vi "Initialise Front Panel.vi"(8 "error in (no error)":errorcluster, 11 "Actor in":refnum<class "Actor.lvclass">) -> (0 "error out":errorcluster, 3 "Actor out":refnum<class "Actor.lvclass">)   [LabVIEW 2015, in "Actor.lvclass"]
uses:
  Actor.lvclass
  Actor.lvclass/Actor.ctl
  Utility/Utility.lvlib
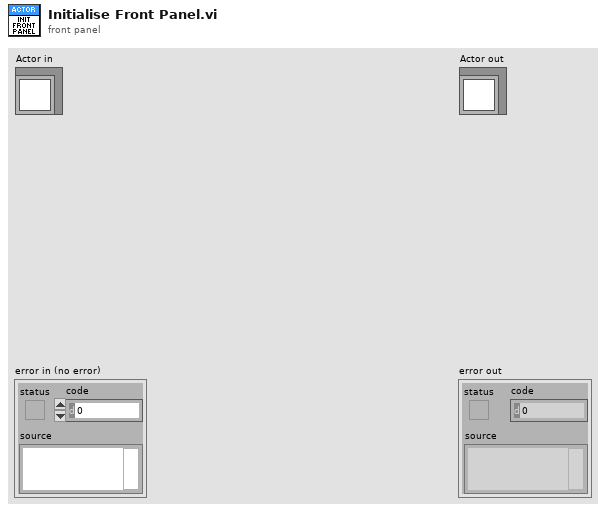
[diagram p1: front panel]
types:
  T1 = enum32{"Invalid", "Standard", "Closed", "Hidden", "Minimized", "Maximized"}
  T2 = typedef "Actor.lvclass/Front Panel State.ctl" = enum32{"Invalid", "Standard", "Closed", "Hidden", "Minimized", "Maximized"}
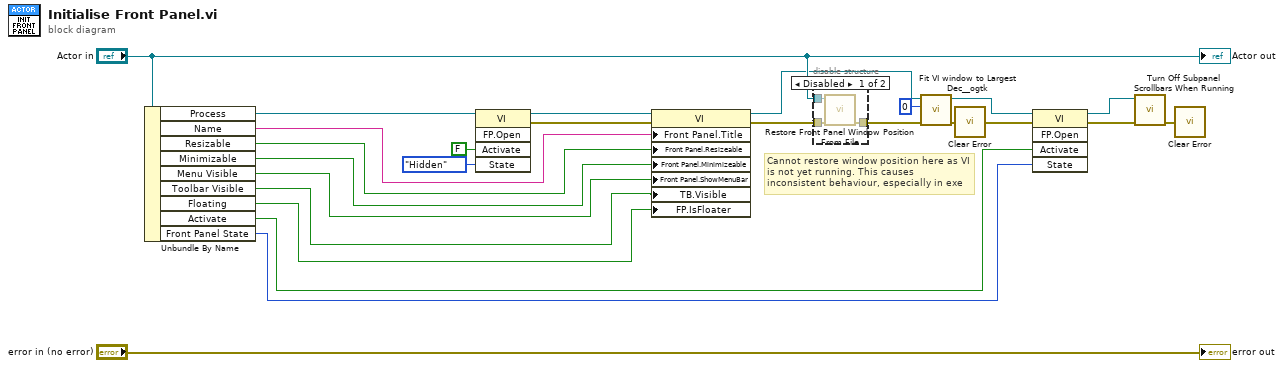
[diagram p0: block diagram]
diagram:
  # "Cannot restore window position here as VI is not yet running. This causes inconsistent behaviour, especially in exe"
  n1 = Unbundle By Name("Actor in") -> ("Process"=w19:refnum<vi>, "Name"=w12:string, "Resizable"=w4:bool, "Minimizable"=w7:bool, "Menu Visible"=w8:bool, "Toolbar Visible"=w1:bool, "Floating"=w3:bool, "Activate"=w5:bool, "Front Panel State"=w25:T2)
  n2 = invoke class="VI" method="FP.Open"(reference=w19, "Activate"=FALSE ("Activate?"), "State"=T1."Hidden") -> (reference out=w14:refnum<vi>, error out=w11:errorcluster)  [unwired: 2 in, 3 out]
  n3 = property class="VI"(reference=w14, error in=w11, "Front Panel.Title"=w12, "Front Panel.Resizeable"=w4, "Front Panel.Minimizeable"=w7, "Front Panel.ShowMenuBar"=w8, "TB.Visible"=w1, "FP.IsFloater"=w3) -> (reference out=w13:refnum<vi>, error out=w2:errorcluster)
  n4 = disable-structure shown="Disabled" {
    disable-tunnel: "Actor in" -> [w28 _]
    disable-tunnel: [w27 w29] -> w17
    disable-tunnel: w2 -> [w26 w29]
    frame Disabled {
      n5 = call "Restore Front Panel Window Position From File.vi"("error in (no error)"=w26, "Actor in"=w28) -> ("error out"=w27:errorcluster)  [unwired: 9 in]
    }
    frame Enabled {
    }
  }
  n6 = call <userlib>:"Fit VI window to Largest Dec__ogtk.vi"("error in (no error)"=w17, "border spacing (2 px)"=0, "VI Ref (calling VI)"=w13) -> ("error out"=w9:errorcluster, "dup VI Ref"=w24:refnum<vi>)  [unwired: 3 in]
  n7 = call "Clear Error.vi"("error in (no error)"=w9) -> ("error out"=w22:errorcluster)
  n8 = invoke class="VI" method="FP.Open"(reference=w24, error in=w22, "Activate"=w5, "State"=w25) -> (reference out=w15:refnum<vi>, error out=w23:errorcluster)  [unwired: 1 in, 3 out]
  n9 = call "Turn Off Subpanel Scrollbars When Running.vi"("error in (no error)"=w23, "VI"=w15) -> ("error out"=w20:errorcluster)  [unwired: 9 in]
  n10 = call "Clear Error.vi"("error in (no error)"=w20) -> ()  [unwired: 1 out]
  "error out" <- "error in (no error)"
  "Actor out" <- "Actor in"
